vi "Incar.vi"() -> ()   [LabVIEW 2025]
uses:
  MsgCluster.ctl
  Incar_state.ctl
panel:
  out "Eventループ終了":bool
  out "consumer1終了した":bool
  out "Data":dbl[](array[numeric])
  out "path 5":string
  out "MsgType 2":T1
  out "path 4":string
  out "Numeric":i32
  out "Consumer2終了した":bool
  out "path 3":string
  out "動画終了フラグ":bool
  out "解析開始フラグ":bool
  out "path 2":string
  out "MsgType":T1
  out "path":string
  out "element 2":T2
  in  "計測開始":bool
  out "element":T2
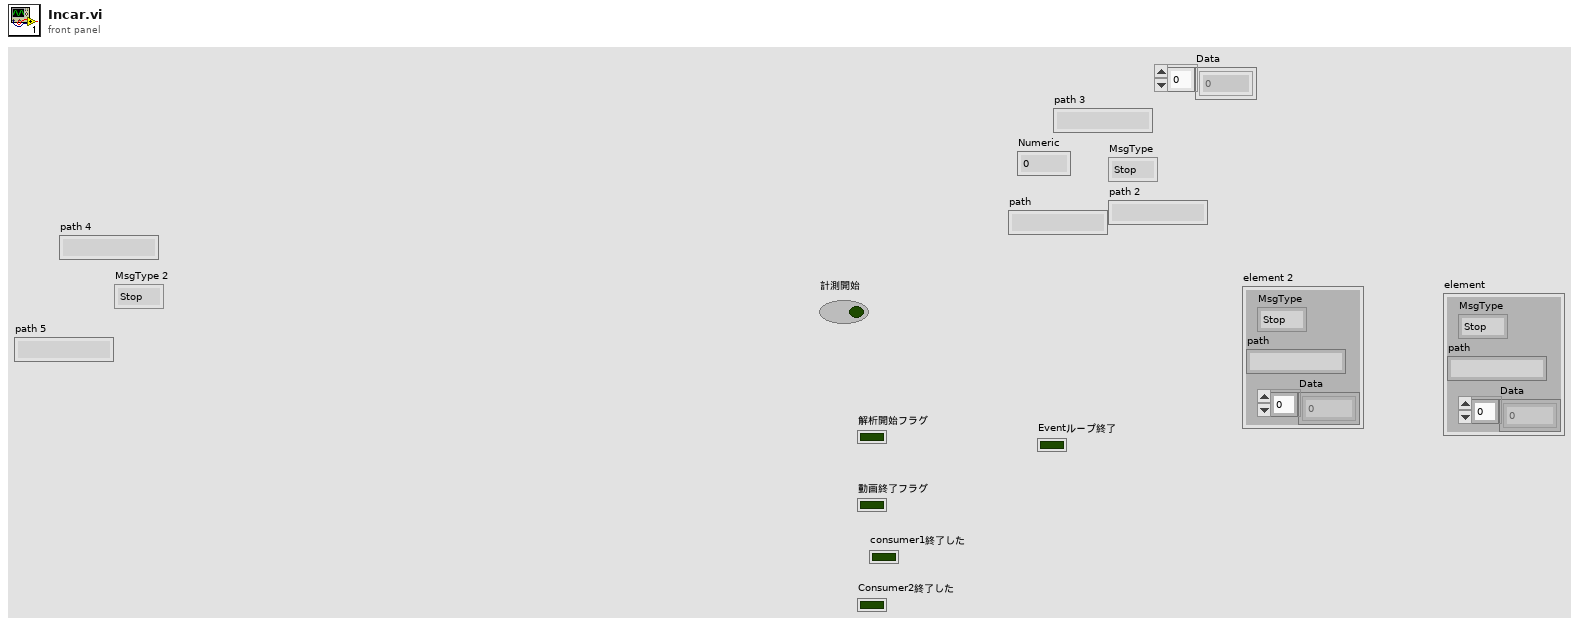
[diagram p1: front panel]
types:
  T1 = typedef "MsgCluster.ctl" = enum16{"Stop", "Start", "Data"}
  T2 = cluster{"MsgType":T1, "path":string, "Data":dbl[]}
  T3 = typedef "Incar_state.ctl" = enum16{"初期化", "待機", "練習", "計測", "解析", "全終了"}
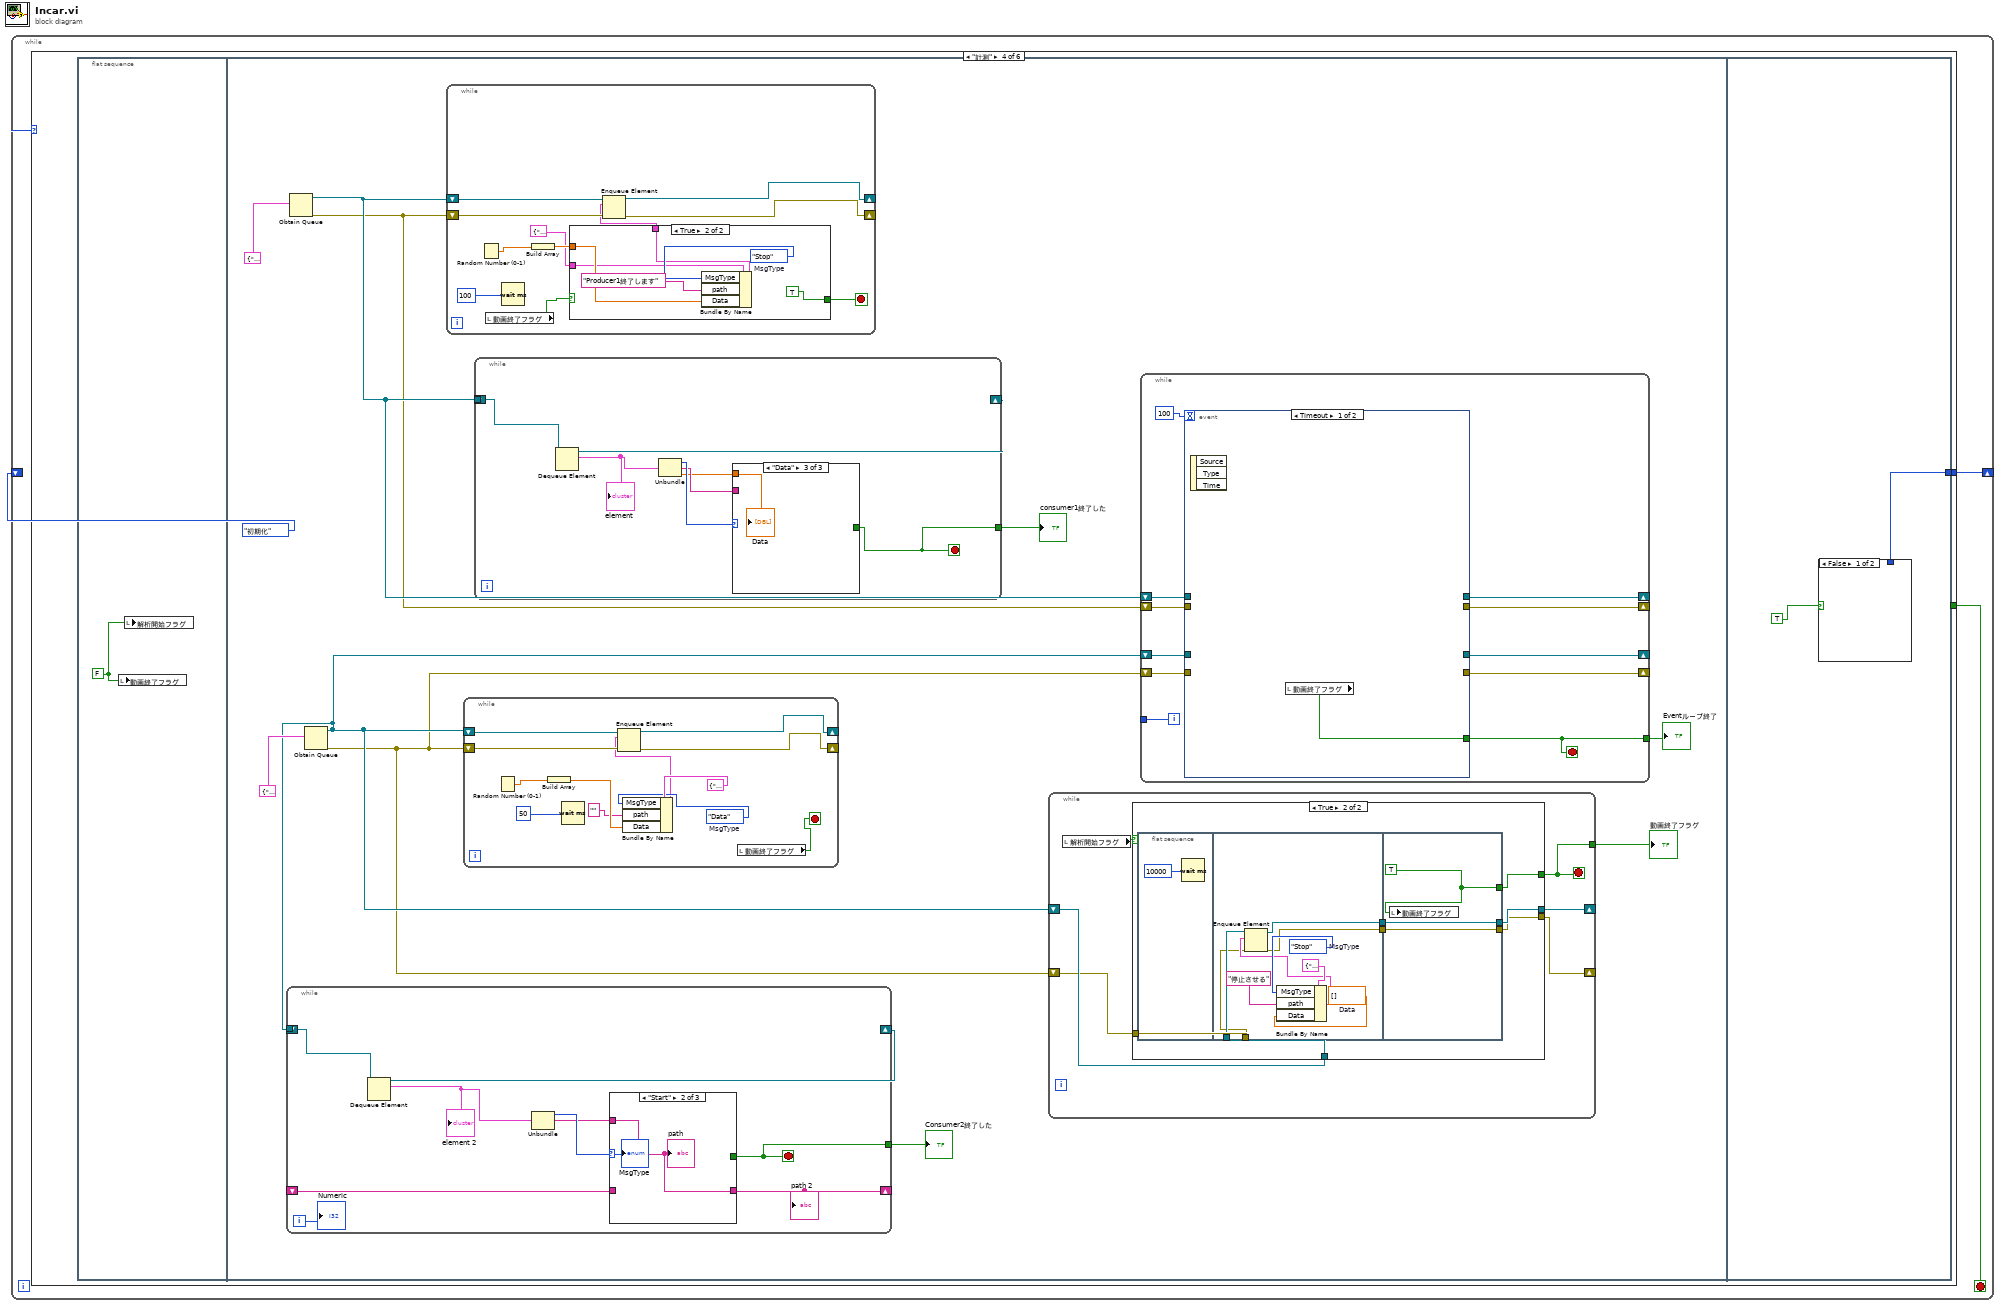
[diagram p0: block diagram]
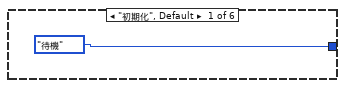
[diagram p2: hidden frame]
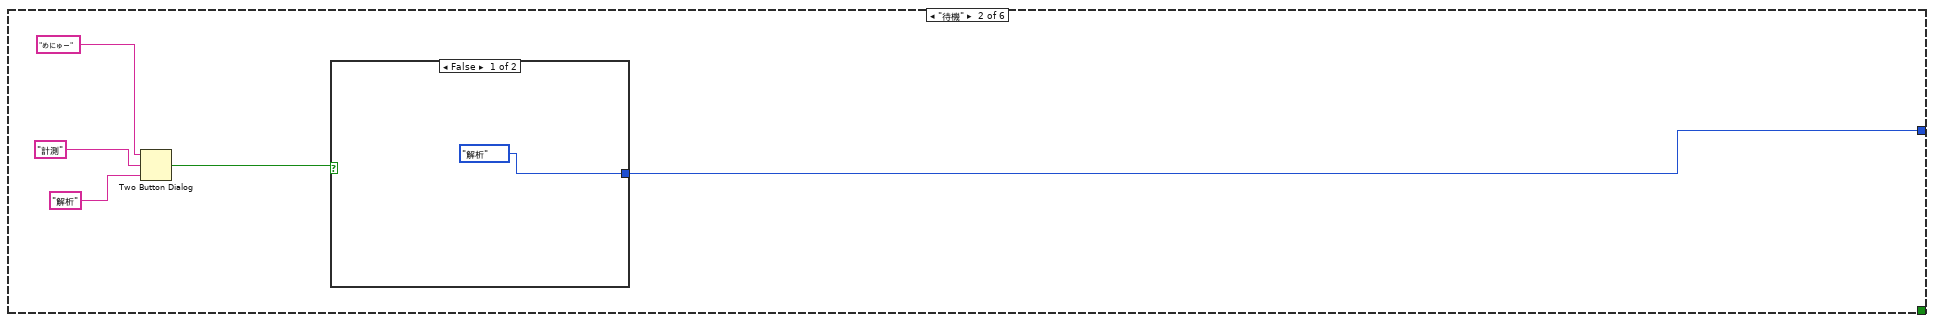
[diagram p3: hidden frame]
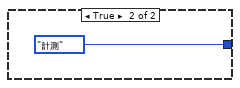
[diagram p4: hidden frame]
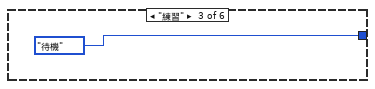
[diagram p5: hidden frame]
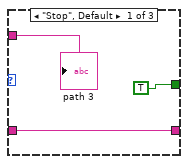
[diagram p7: hidden frame]
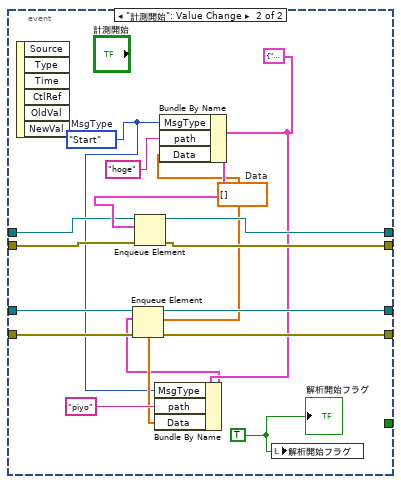
[diagram p9: hidden frame]
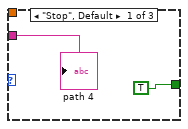
[diagram p10: hidden frame]
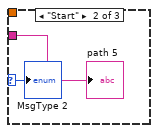
[diagram p11: hidden frame]
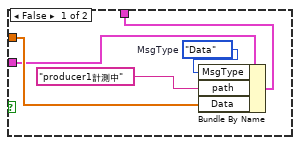
[diagram p12: hidden frame]
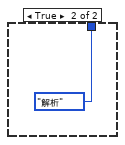
[diagram p13: hidden frame]
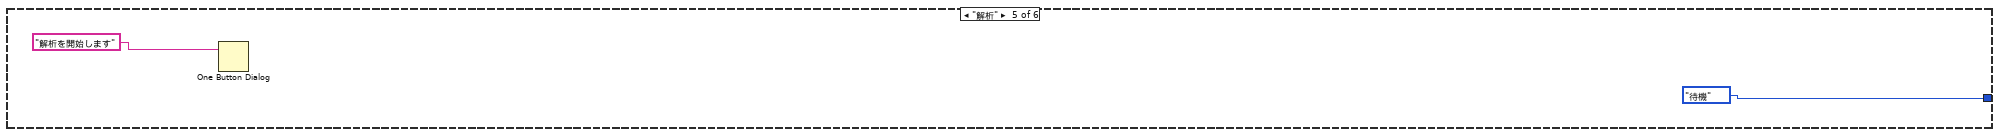
[diagram p14: hidden frame]
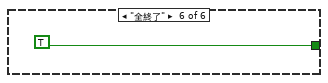
[diagram p15: hidden frame]
diagram:
  n1 = while {
    shift-right: [w3] -> _
    shift-left: Incar_state."初期化" -> [w4]
    stop <- w2 stop-if-true
    n2 = case shown="\"計測\"" w4 {
      tunnel: [Incar_state."待機" w7 Incar_state."待機" w14 Incar_state."待機" _] -> w3
      tunnel: [_ _ _ _ _ TRUE] -> w2
      frame "初期化", Default {
      }
      frame "待機" {
        n3 = Two Button Dialog(message="めにゅー", 1:"解析", 2:"計測") -> (T button?=w8:bool)
        n4 = case shown="False" w8 {
          tunnel: [Incar_state."解析" Incar_state."計測"] -> w7
          frame False {
          }
          frame True {
          }
        }
      }
      frame "練習" {
      }
      frame "計測" {
        n5 = flat-sequence {
          tunnel: [w142] -> w14
          frame #0 {
            w15 = FALSE
            n6 = local write "動画終了フラグ"(w15) -> ()
            n7 = local write "解析開始フラグ"(w15) -> ()
          }
          frame #1 {
            n8 = Obtain Queue(element data type=T2 {"MsgType"=enum."Stop", "path"="", "Data"=[]}) -> (queue out=w24:refnum<queue>, error out=w23:errorcluster)  [unwired: 4 in, 1 out]
            n9 = Obtain Queue(element data type=T2 {"MsgType"=enum."Stop", "path"="", "Data"=[]}) -> (queue out=w21:refnum<queue>, error out=w20:errorcluster)  [unwired: 4 in, 1 out]
            n10 = while {
              tunnel: w21 -> [w60]
              shift-right: [w59] -> _
              shift-left: _ -> [_]
              shift-right: [w54] -> _
              shift-left: _ -> [w56]
              tunnel: [w52] -> w18
              i -> [w53]
              stop <- w52 stop-if-true
              n11 = Dequeue Element(queue=w60) -> (queue out=w59:refnum<queue>, element=w58:T2)  [unwired: 2 in, 2 out]
              "element 2" <- w58
              n12 = Unbundle(w58) -> ("MsgType"=w57:T1, "path"=w55:string)  [unwired: 1 out]
              n13 = case shown="\"Start\"" w57 {
                selector: w57 -> [_ w64 _]
                tunnel: w56 -> [w63 _ w66]
                tunnel: w55 -> [w62 w65 _]
                tunnel: [w63 w65 w66] -> w54
                tunnel: [TRUE _ _] -> w52
                frame "Stop", Default {
                  "path 3" <- w62
                }
                frame "Start" {
                  "path" <- w65
                  "MsgType" <- w64
                }
                frame "Data" {
                }
              }
              "path 2" <- w54
              "Numeric" <- w53
            }
            "Consumer2終了した" <- w18
            n14 = while {
              shift-right: [w126] -> _
              shift-left: w24 -> [w128]
              shift-right: [w122] -> _
              shift-left: w23 -> [w127]
              stop <- w119 stop-if-true
              n15 = Random Number (0-1)() -> (number: 0 to 1=w125:dbl)
              n16 = local read "動画終了フラグ"() -> (w121:bool)
              n17 = Wait (ms)(milliseconds to wait=100) -> ()  [unwired: 1 out]
              n18 = Build Array(w125) -> (w124:dbl[])
              n19 = case shown="True" w121 {
                tunnel: w124 -> [w132 w140]
                tunnel: [w130 w137] -> w123
                tunnel: T2 {"MsgType"=enum."Stop", "path"="", "Data"=[]} -> [w131 w136]
                tunnel: [_ TRUE] -> w119
                frame False {
                  w133 = MsgCluster."Data"  # MsgType
                  n20 = Bundle By Name(cluster=w131, "MsgType"=w133, "path"="producer1計測中", "Data"=w132) -> (w130:T2)
                }
                frame True {
                  w138 = MsgCluster."Stop"  # MsgType
                  n21 = Bundle By Name(cluster=w136, "MsgType"=w138, "path"="Producer1終了します", "Data"=w140) -> (w137:T2)
                }
              }
              n22 = Enqueue Element(queue=w128, element=w123, error in (no error)=w127) -> (queue out=w126:refnum<queue>, error out=w122:errorcluster)  [unwired: 1 in, 1 out]
            }
            n23 = while {
              shift-right: [w75] -> _
              shift-left: w21 -> [w77]
              shift-right: [w68] -> _
              shift-left: w20 -> [w76]
              stop <- w67 stop-if-true
              w70 = MsgCluster."Data"  # MsgType
              n24 = Random Number (0-1)() -> (number: 0 to 1=w74:dbl)
              n25 = Build Array(w74) -> (w72:dbl[])
              n26 = Wait (ms)(milliseconds to wait=50) -> ()  [unwired: 1 out]
              n27 = Bundle By Name(cluster=T2 {"MsgType"=enum."Stop", "path"="", "Data"=[]}, "MsgType"=w70, "path"="", "Data"=w72) -> (w69:T2)
              n28 = Enqueue Element(queue=w77, element=w69, error in (no error)=w76) -> (queue out=w75:refnum<queue>, error out=w68:errorcluster)  [unwired: 1 in, 1 out]
              n29 = local read "動画終了フラグ"() -> (w67:bool)
            }
            n30 = while {
              tunnel: w24 -> [w113]
              shift-right: [w112] -> _
              shift-left: _ -> [_]
              tunnel: [w107] -> w19
              stop <- w107 stop-if-true
              n31 = Dequeue Element(queue=w113) -> (queue out=w112:refnum<queue>, element=w109:T2)  [unwired: 2 in, 2 out]
              "element" <- w109
              n32 = Unbundle(w109) -> ("MsgType"=w111:T1, "path"=w110:string, "Data"=w108:dbl[])
              n33 = case shown="\"Data\"" w111 {
                selector: w111 -> [_ w116 _]
                tunnel: w110 -> [w115 w117 _]
                tunnel: [TRUE _ _] -> w107
                tunnel: w108 -> [_ _ w118]
                frame "Stop", Default {
                  "path 4" <- w115
                }
                frame "Start" {
                  "path 5" <- w117
                  "MsgType 2" <- w116
                }
                frame "Data" {
                  "Data" <- w118
                }
              }
            }
            "consumer1終了した" <- w19
            n34 = while {
              shift-right: [w29] -> _
              shift-left: w21 -> [w30]
              shift-right: [w27] -> _
              shift-left: w20 -> [w28]
              tunnel: [w26] -> w17
              stop <- w26 stop-if-true
              n35 = local read "解析開始フラグ"() -> (w31:bool)
              n36 = case shown="True" w31 {
                tunnel: [_ w38] -> w26
                tunnel: w30 -> [_ w37]
                tunnel: [_ w36] -> w29
                tunnel: w28 -> [_ w35]
                tunnel: [_ w34] -> w27
                frame False {
                }
                frame True {
                  n37 = flat-sequence {
                    tunnel: w37 -> [w48]
                    tunnel: w35 -> [w41]
                    tunnel: [w47] -> w33
                    tunnel: [w40] -> w32
                    tunnel: [w50] -> w34
                    tunnel: [w51] -> w36
                    tunnel: [w49] -> w38
                    tunnel: w33 -> [w51]
                    tunnel: w32 -> [w50]
                    frame #0 {
                      n38 = Wait (ms)(milliseconds to wait=10000) -> ()  [unwired: 1 out]
                    }
                    frame #1 {
                      w43 = MsgCluster."Stop"  # MsgType
                      w44 = dbl[] []  # Data
                      n39 = Bundle By Name(cluster=T2 {"MsgType"=enum."Stop", "path"="", "Data"=[]}, "MsgType"=w43, "path"="停止させる", "Data"=w44) -> (w42:T2)
                      n40 = Enqueue Element(queue=w48, element=w42, error in (no error)=w41) -> (queue out=w47:refnum<queue>, error out=w40:errorcluster)  [unwired: 1 in, 1 out]
                    }
                    frame #2 {
                      w49 = TRUE
                      n41 = local write "動画終了フラグ"(w49) -> ()
                    }
                  }
                }
              }
            }
            "動画終了フラグ" <- w17
            n42 = while {
              shift-right: [w86] -> _
              shift-left: w24 -> [w89]
              tunnel: [w87] -> _
              shift-right: [w85] -> _
              shift-left: w23 -> [w88]
              shift-right: [w81] -> _
              shift-left: w20 -> [w83]
              shift-right: [w82] -> _
              shift-left: w21 -> [w84]
              tunnel: [w80] -> w16
              i -> [w87]
              stop <- w80 stop-if-true
              n43 = event shown="[0] Timeout" {
                selector: _ -> [_ _]
                dyn-events: _ -> [_ _]
                timeout: 100 -> [_ _]
                tunnel: w89 -> [_ w104]
                tunnel: w88 -> [_ w103]
                tunnel: [_ w102] -> w86
                tunnel: [_ w101] -> w85
                tunnel: w84 -> [_ w100]
                tunnel: w83 -> [_ w99]
                tunnel: [_ w98] -> w82
                tunnel: [_ w97] -> w81
                tunnel: [w90 _] -> w80
                event Timeout {
                  n44 = event-data() -> ()  [unwired: 1 in, 3 out]
                  n45 = local read "動画終了フラグ"() -> (w90:bool)
                }
                event "計測開始": Value Change {
                  w91 = TRUE
                  w96 = T2 {"MsgType"=enum."Stop", "path"="", "Data"=[]}
                  w94 = dbl[] []  # Data
                  w93 = MsgCluster."Start"  # MsgType
                  n46 = event-data() -> ()  [unwired: 1 in, 6 out]
                  n47 = Bundle By Name(cluster=w96, "MsgType"=w93, "path"="piyo", "Data"=w94) -> (w92:T2)
                  n48 = Enqueue Element(queue=w100, element=w92, error in (no error)=w99) -> (queue out=w98:refnum<queue>, error out=w97:errorcluster)  [unwired: 1 in, 1 out]
                  n49 = Bundle By Name(cluster=w96, "MsgType"=w93, "path"="hoge", "Data"=w94) -> (w105:T2)
                  n50 = Enqueue Element(queue=w104, element=w105, error in (no error)=w103) -> (queue out=w102:refnum<queue>, error out=w101:errorcluster)  [unwired: 1 in, 1 out]
                  n51 = local write "解析開始フラグ"(w91) -> ()
                  "解析開始フラグ" <- w91
                }
              }
            }
            "Eventループ終了" <- w16
          }
          frame #2 {
            n52 = case shown="False" TRUE {
              tunnel: [_ Incar_state."解析"] -> w142
              frame False {
              }
              frame True {
              }
            }
          }
        }
      }
      frame "解析" {
        n53 = One Button Dialog(message="解析を開始します") -> ()  [unwired: 1 in, 1 out]
      }
      frame "全終了" {
      }
    }
  }
